vi "Construct.vi"(7 "Buffer":T1=50, 8 "Error in (no error)":errorcluster, 9 "Array LogFilterInterface in":refnum<class "LogFilterInterface.lvclass">[](array[class]), 10 "LogWriterInterface in":refnum<class "LogWriterInterface.lvclass">) -> (0 "Error out":errorcluster, 3 "Log out":refnum<class "Log.lvclass">)   [LabVIEW 2011, in "Log.lvclass"]
uses:
  Log.lvclass
  Writer/LogWriterInterface/LogWriterInterface.lvclass
  Filter/LogFilterInterface/LogFilterInterface.lvclass
  Buffer.ctl
  Writer/LogWriterMock/LogWriterMock.lvclass
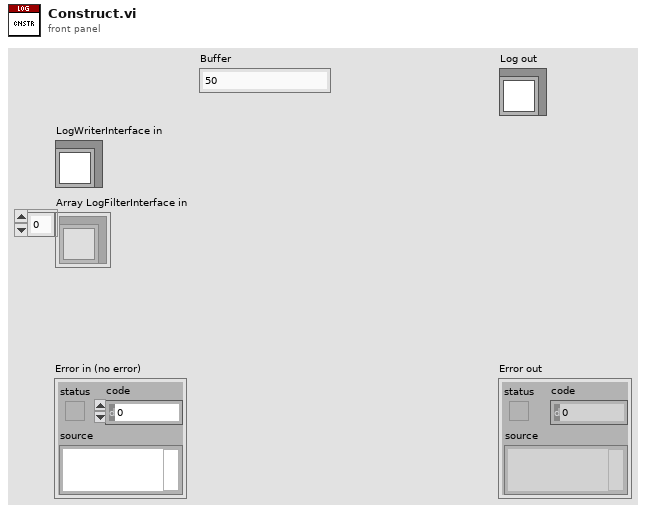
[diagram p1: front panel]
types:
  T1 = typedef "Log.lvclass/Buffer.ctl" = u32
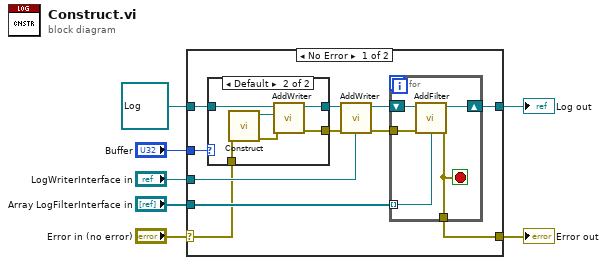
[diagram p0: block diagram]
diagram:
  n1 = case shown="No Error" "Error in (no error)" {
    selector: "Error in (no error)" -> [w9 w33]
    tunnel: [w13 w33] -> w6
    tunnel: [w16 w32] -> w5
    tunnel: refnum<class "Log.lvclass"> refnum ("Log in") -> [w12 w32]
    tunnel: "LogWriterInterface in" -> [w18 _]
    tunnel: "Array LogFilterInterface in" -> [w15 _]
    tunnel: "Buffer" -> [w8 _]
    frame No Error {
      n2 = case shown="Default" w8 {
        tunnel: w12 -> [w19 w23]
        tunnel: [w19 w26] -> w11
        tunnel: [w20 w25] -> w10
        tunnel: w9 -> [w20 w21]
        frame 0 {
        }
        frame Default {
          n3 = call "Construct.vi"("Error in (no error)"=w21) -> ("Error out"=w22:errorcluster, "LogWriterMock out"=w24:refnum<class "LogWriterMock.lvclass">)  [unwired: 9 in]
          n4 = call "AddWriter.vi"("Error in (no error)"=w22, "LogWriterInterface in"=w24, "Log in"=w23) -> ("Error out"=w25:errorcluster, "Log out"=w26:refnum<class "Log.lvclass">)  [unwired: 7 in]
        }
      }
      n5 = call "AddWriter.vi"("Error in (no error)"=w10, "LogWriterInterface in"=w18, "Log in"=w11) -> ("Error out"=w14:errorcluster, "Log out"=w17:refnum<class "Log.lvclass">)  [unwired: 7 in]
      n6 = for {
        shift-right: [w30] -> w16
        shift-left: w17 -> [w31]
        tunnel: w15 -> [w29] mode=indexing
        tunnel: w14 -> [w28]
        tunnel: [w27] -> w13
        stop <- w27 stop-if-true
        n7 = call "AddFilter.vi"("Error in (no error)"=w28, "LogFilterInterface in"=w29, "Log in"=w31) -> ("Error out"=w27:errorcluster, "Log out"=w30:refnum<class "Log.lvclass">)  [unwired: 7 in]
      }
    }
    frame Error {
    }
  }
  "Error out" <- w6
  "Log out" <- w5
